vi "FF_BellShapeFun.vi"(3 "Invert(F)":bool, 4 "(r)adius":dbl, 5 "(A)mplitude":dbl, 6 "x":dbl) -> (1 "y":dbl)   [LabVIEW 2016, in "ForceField.lvclass"]
uses:
  ForceField.lvclass
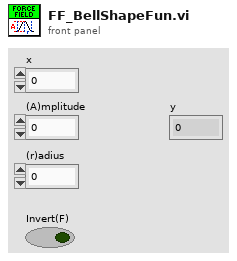
[diagram p1: front panel]
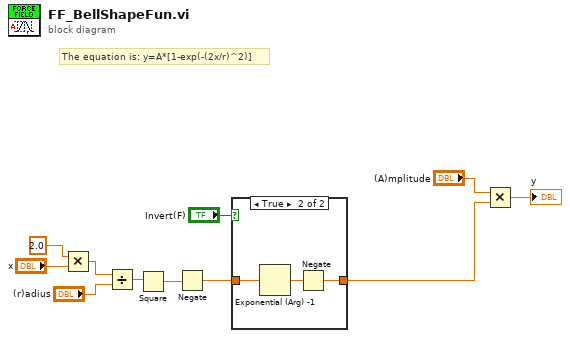
[diagram p0: block diagram]
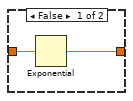
[diagram p2: hidden frame]
diagram:
  # "The equation is: y=A*[1-exp(-(2x/r)^2)]"
  n1 = Multiply(x=2.0, y="x") -> (x*y=w9:dbl)
  n2 = Divide(x=w9, y="(r)adius") -> (x/y=w7:dbl)
  n3 = Square(x=w7) -> (x^2=w6:dbl)
  n4 = Negate(x=w6) -> (-x=w5:dbl)
  n5 = case shown="True" "Invert(F)" {
    tunnel: w5 -> [w13 w16]
    tunnel: [w12 w14] -> w2
    frame False {
      n6 = Exponential(1:w13) -> (0:w12:dbl)
    }
    frame True {
      n7 = Exponential (Arg) -1(1:w16) -> (0:w15:dbl)
      n8 = Negate(x=w15) -> (-x=w14:dbl)
    }
  }
  n9 = Multiply(x="(A)mplitude", y=w2) -> (x*y=→"y":dbl)
